vi "DiffOdometry_Update.vi"(6 "Reset Pose":T1={"TRANSLATION"={"X"=0.0, "Y"=0.0}, "ROTATION"={"VALUE"=0.0, "COS"=1.0, "SIN"=0.0}}, 8 "Reset":bool, 9 "Heading":T3={"VALUE"=0.0, "COS"=1.0, "SIN"=0.0}, 10 "RightDistance":dbl, 11 "LeftDistance":dbl) -> (3 "CurrentRelativePose":T1)   [LabVIEW 2019, in "Trajectory_Library.lvlib"]
doc: "SubVI for differential drive odometry. Odometry allows you to track the robot's position on the field over the course of a match using readings from 2 encoders and a gyroscope.\n\nTeams can use odometry during the autonomous period for complex tasks like path following. Furthermore, odometry can be used for latency compensation when using computer-vision systems.\n\nUpdates the robot position on the field using distance measurements from encoders. This method is more numerically accurate than using velocities to integrate the pose and is also advantageous for teams that are using lower CPR encoders.\n\nThis implementation slightly differs from the WPILIB C++/Java. The constructor, Update and Reset functions are incorporated into this single routine. There is no need to reset encoders or gyros. This routine compensates by remembering the values at reset. An optional \"Initial POSE\" can be specified to allow this routine to calculate absolute position. If not specified the position is relative to the position at reset. More than one instance of this can be used if needed. One instance could track absolute field position while another instance can track relative position for executing a trajectory.\n\nParameters:\n - Left distance -- Left wheel encoder distance (meters)\n - Right distance -- Right wheel encodeer distance (meters)\n - Heading - Robot gyroscope reading\n - Reset - When set, this resets the remembered left, right distance and gyroscope values, and sets the current pose to the initial pose. \n - Reset Pose - (Optional) When reset is TRUE this pose is used to set the current robot pose. (If the inital pose is zero or not present, the result will be a relative pose. If the reset pose is the absolute field pose, then the result current pose will be absolute.)\n\nResults:\n - currentRelativePose - The new pose of the robot. (If the initial pose is absolute, this will be an absolute pose.)"
uses:
  Trajectory_Library.lvlib
  POSE2D.ctl
  TRANSLATION2D.ctl
  ROTATION2D.ctl
  Rotation_UnaryMinus.vi
  Rotation_RotateBy.vi
  Rotation_CreateAngle.vi
  Rotation_CreateXY.vi
  Util_CalcDist.vi
  <vilib>/Rock Robotics/SystemInterfaces/NetworkCommunication/NetComm_UsageReport_ResourceType.ctl
  Util_LibraryGlobals.vi
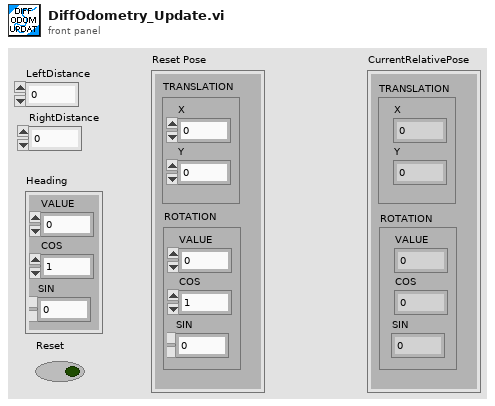
[diagram p1: front panel]
types:
  T1 = typedef "Trajectory_Library.lvlib/POSE2D.ctl" = cluster{"TRANSLATION":T2, "ROTATION":T3}
  T2 = typedef "Trajectory_Library.lvlib/TRANSLATION2D.ctl" = cluster{"X":dbl, "Y":dbl}
  T3 = typedef "Trajectory_Library.lvlib/ROTATION2D.ctl" = cluster{"VALUE":dbl, "COS":dbl, "SIN":dbl}
  T4 = typedef "NetComm_UsageReport_ResourceType.ctl" = enum8{"Controller", "Module", "Language", "CANPlugin", "Accelerometer", "ADXL345", "AnalogChannel", "AnalogTrigger", "AnalogTriggerOutput", "CANJaguar", "Compressor", "Counter", "Dashboard", "DigitalInput", "DigitalOutput", "DriverStationCIO", "DriverStationEIO", "DriverStationLCD", "Encoder", "GearTooth", "Gyro", "I2C", "Framework", "Jaguar", "Joystick", "Kinect", "KinectStick", "PIDController", "Preferences", "PWM", "Relay", "RobotDrive", "SerialPort", "Servo", "Solenoid", "SPI", "Task", "Ultrasonic", "Victor", "Button", "Command", "AxisCamera", "PCVideoServer", "SmartDashboard", "Talon", "HiTechnicColorSensor", "HiTechnicAccel", "HiTechnicCompass", "SRF08", "AnalogOutput", "Victor SP", "Talon SRX", "CAN Talon SRX", "ADXL362 Accel", "ADXRS450 Gyro", "Rev SPARK", "Mindsensors SD540", "Digital Filter", "ADIS16448", "PDP", "PCM", "PigeonIMU", "Nidec Brushless", "CTRE CANifier", "CTRE TalonFX", "CTRE Future 1", "CTRE Future 2", "CTRE Future 3", "CTRE Future 4", "CTRE Future 5", "CTRE Future 6", "Linear Filter", "Xbox Controller", "USB Camera", "NavX", "Pixy", "Pixy2", "ScanseSweep", "Shuffleboard", "CAN", "Digilent DMC60", "PWM Victor SPX", "Rev SPARK MAX PWM", "Rev SPARK MAX CAN", "ADIS16470", "PIDController2", "ProfiledPIDController", "Kinematics", "Odometry", "Units", "Trapezoid Profile", "DutyCycle", "Addressable LEDs", "Fusion Venom"}
  T5 = typedef "Trajectory_Library.lvlib/TWIST2D.ctl" = cluster{"dX":dbl, "dY":dbl, "dTHETA":dbl}
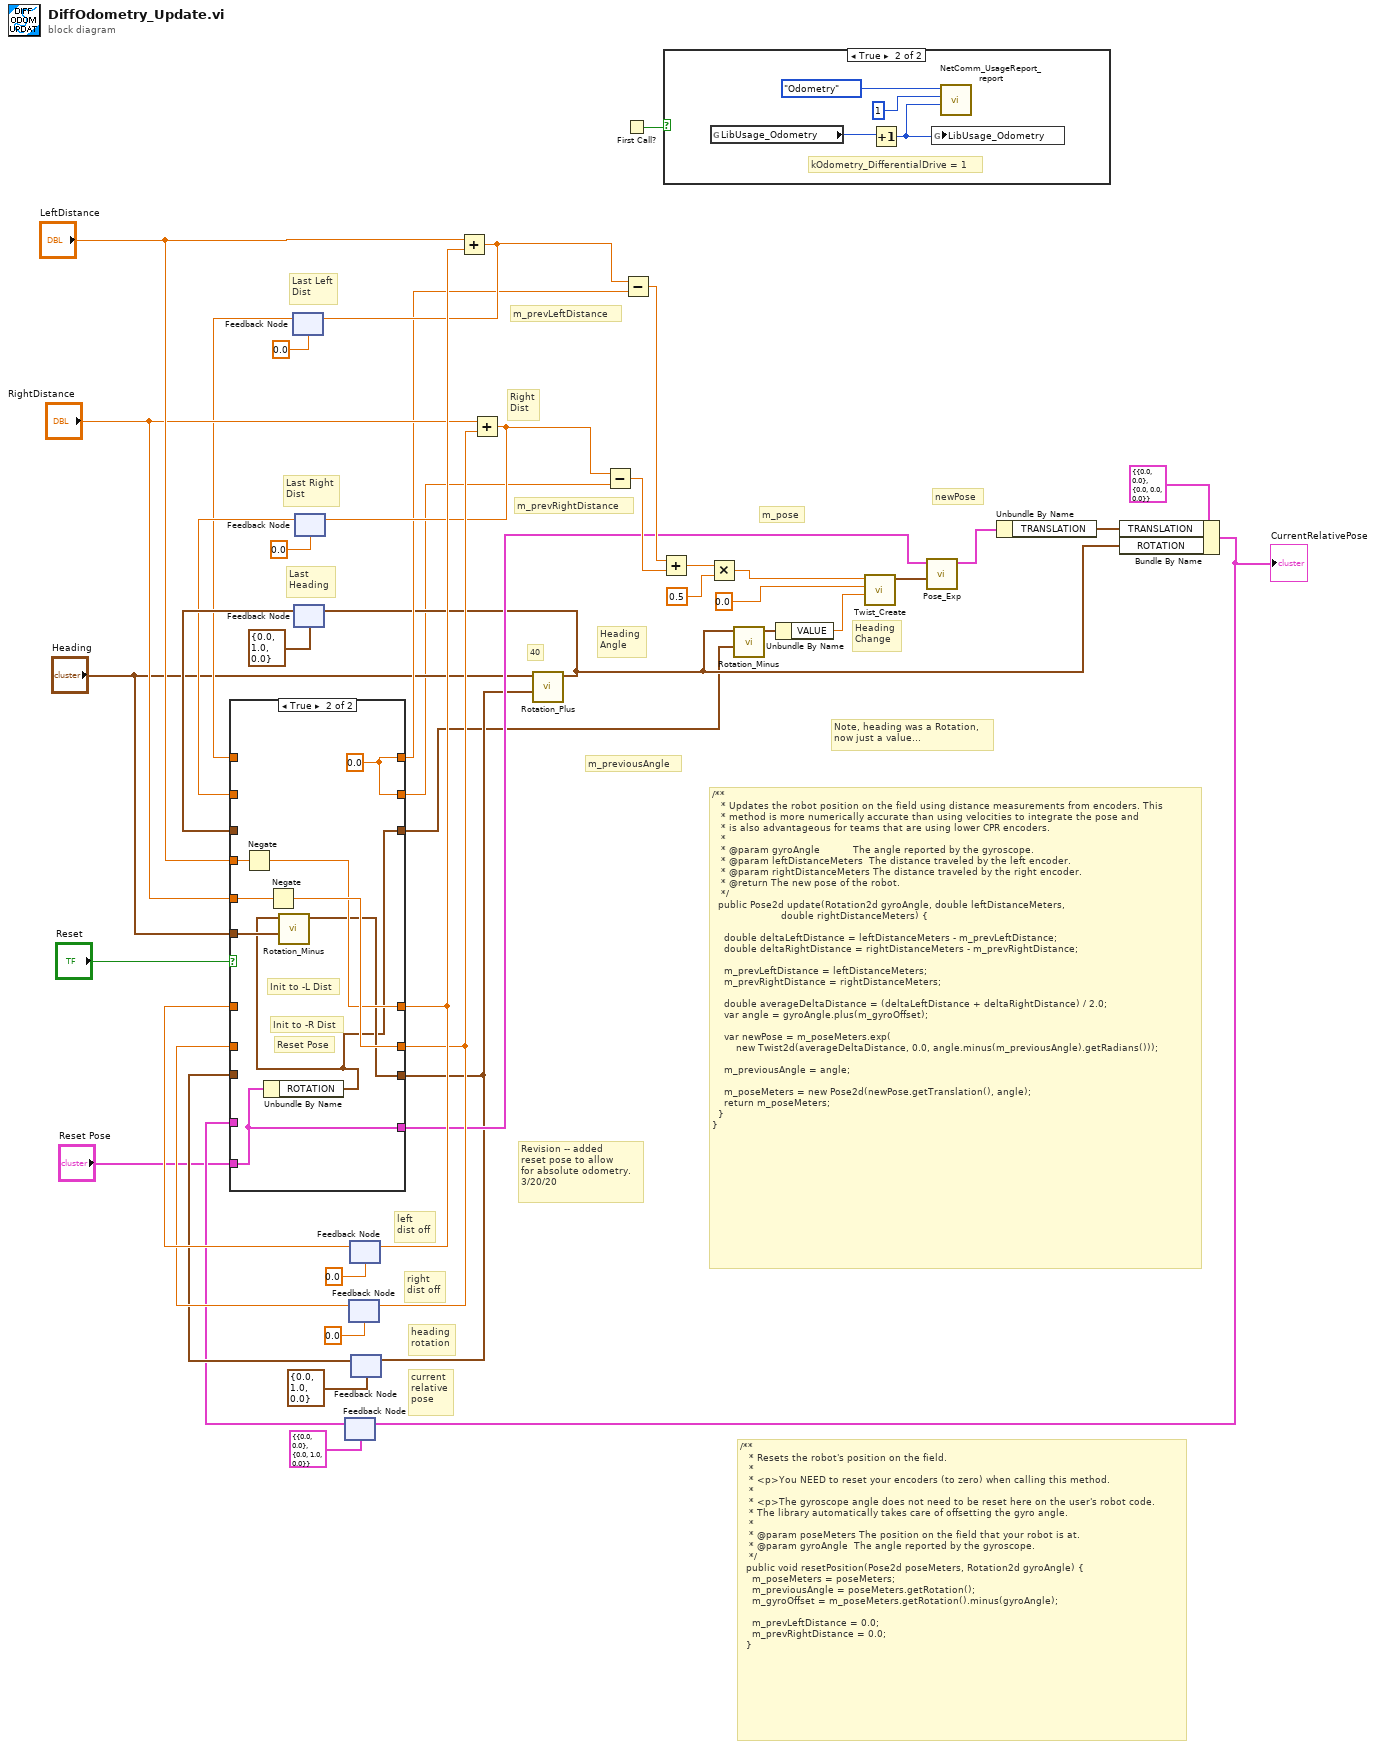
[diagram p0: block diagram]
diagram:
  # "Revision -- added\nreset pose to allow\nfor absolute odometry.\n3/20/20"
  # "40"
  # "left\ndist off"
  # "right\ndist off"
  # "heading\nrotation"
  # "current \nrelative\npose"
  # "/**\n   * Resets the robot's position on the field.\n   *\n   * <p>You NEED to reset your encoders (to zero) when calling this method.\n   *\n   * <p>The gyroscope angle does not need to be reset here on the user's robot code.\n   * The library automatically takes care of offsetting the gyro angle.\n   *\n   * @param poseMeters The position on the field that your robot is at.\n   * @param gyroAngle  The angle reported by the gyroscope.\n   */\n  public void resetPosition(Pose2d poseMeters, Rotation2d gyroAngle) {\n    m_poseMeters = poseMeters;\n    m_previousAngle = poseMeters.getRotation();\n    m_gyroOffset = m_poseMeters.getRotation().minus(gyroAngle);\n\n    m_prevLeftDistance = 0.0;\n    m_prevRightDistance = 0.0;\n  }"
  # "Heading\nChange"
  # "Note, heading was a Rotation,\nnow just a value..."
  # "Last\nHeading"
  # "Last Right\nDist"
  # "Last Left\nDist"
  # "Right\nDist"
  # "/**\n   * Updates the robot position on the field using distance measurements from encoders. This\n   * method is more numerically accurate than using velocities to integrate the pose and\n   * is also advantageous for teams that are using lower CPR encoders.\n   *\n   * @param gyroAngle           The angle reported by the gyroscope.\n   * @param leftDistanceMeters  The distance traveled by the left encoder.\n   * @param rightDistanceMeters The distance traveled by the right encoder.\n   * @return The new pose of the robot.\n   */\n  public Pose2d update(Rotation2d gyroAngle, double leftDistanceMeters,\n                       double rightDistanceMeters) {\n\n    double deltaLeftDistance = leftDistanceMeters - m_prevLeftDistance;\n    double deltaRightDistance = rightDistanceMeters - m_prevRightDistance;\n\n    m_prevLeftDistance = leftDistanceMeters;\n    m_prevRightDistance = rightDistanceMeters;\n\n    double averageDeltaDistance = (deltaLeftDistance + deltaRightDistance) / 2.0;\n    var angle = gyroAngle.plus(m_gyroOffset);\n\n    var newPose = m_poseMeters.exp(\n        new Twist2d(averageDeltaDistance, 0.0, angle.minus(m_previousAngle).getRadians()));\n\n    m_previousAngle = angle;\n\n    m_poseMeters = new Pose2d(newPose.getTranslation(), angle);\n    return m_poseMeters;\n  }\n}"
  # "newPose"
  # "Heading\nAngle"
  # "m_prevRightDistance"
  # "m_prevLeftDistance"
  # "m_previousAngle"
  # "m_pose"
  n1 = feedback #1(0.0 ("LeftDistance")) -> (w16:dbl)
  n2 = feedback #2(T3 {"VALUE"=0.0, "COS"=1.0, "SIN"=0.0} ("ROTATION")) -> (w19:T3)
  n3 = feedback #3(0.0 ("RightDistance")) -> (w18:dbl)
  n4 = feedback #4(T1 {"TRANSLATION"={"X"=0.0, "Y"=0.0}, "ROTATION"={"VALUE"=0.0, "COS"=1.0, "SIN"=0.0}} ("POSE")) -> (w21:T1)
  n5 = feedback #5(0.0 ("LeftDistance")) -> (w35:dbl)
  n6 = feedback #6(0.0 ("LeftDistance")) -> (w36:dbl)
  n7 = feedback #7(T3 {"VALUE"=0.0, "COS"=1.0, "SIN"=0.0} ("ROTATION")) -> (w34:T3)
  n8 = case shown="True" "Reset" {
    tunnel: "Heading" -> [_ w54]
    tunnel: "RightDistance" -> [_ w58]
    tunnel: "LeftDistance" -> [_ w59]
    tunnel: [w50 w56] -> w30
    tunnel: [w49 w57] -> w26
    tunnel: [w48 w55] -> w6
    tunnel: w36 -> [w50 _]
    tunnel: w35 -> [w49 _]
    tunnel: w34 -> [w48 _]
    tunnel: [w47 w51] -> w20
    tunnel: w21 -> [w47 _]
    tunnel: w19 -> [w46 _]
    tunnel: [w46 w53] -> w4
    tunnel: w18 -> [w45 _]
    tunnel: [w45 w52] -> w3
    tunnel: [w44 w52] -> w17
    tunnel: w16 -> [w44 _]
    tunnel: "Reset Pose" -> [_ w51]
    frame False {
      # "Last Left Dist"
      # "Last Right Dist"
      # "Last Heading"
      # "(-) Left Dist at Reset"
      # "(-) Right Dist at Reset"
      # "Heading at Reset"
      # "Saved Relative POSE"
    }
    frame True {
      w52 = 0.0 ("LeftDistance")
      # "Init to -L Dist"
      # "Init to -R Dist"
      # "Reset Pose"
      n9 = Negate(x=w59) -> (-x=w56:dbl)
      n10 = Unbundle By Name(w51) -> ("ROTATION"=w53:T3)
      n11 = Negate(x=w58) -> (-x=w57:dbl)
      n12 = call "Rotation_Minus.vi"("other ROTATION"=w54, "in ROTATION"=w53) -> ("out ROTATION"=w55:T3)  [unwired: 9 in]
    }
  }
  n13 = feedback-in #5(w26) -> ()
  n14 = feedback-in #6(w30) -> ()
  n15 = feedback-in #7(w6) -> ()
  n16 = Add(x="LeftDistance", y=w30) -> (x+y=w28:dbl)
  n17 = feedback-in #1(w28) -> ()
  n18 = Add(x="RightDistance", y=w26) -> (x+y=w25:dbl)
  n19 = feedback-in #3(w25) -> ()
  n20 = call "Rotation_Plus.vi"("other ROTATION"=w6, "in ROTATION"="Heading") -> ("out ROTATION"=w5:T3)  [unwired: 9 in]
  n21 = feedback-in #2(w5) -> ()
  n22 = Subtract(x=w25, y=w3) -> (x-y=w42:dbl)
  n23 = First Call?() -> (First Call?: T/F=w1:bool)
  n24 = Subtract(x=w28, y=w17) -> (x-y=w43:dbl)
  n25 = Add(x=w43, y=w42) -> (x+y=w41:dbl)
  n26 = case shown="True" w1 {
    frame False {
    }
    frame True {
      # "kOdometry_DifferentialDrive = 1"
      n27 = global read "Util_LibraryGlobals.vi" "LibUsage_Odometry"() -> (w62:i32)
      n28 = Increment(x=w62) -> (x+1=w61:i32)
      n29 = global write "Util_LibraryGlobals.vi" "LibUsage_Odometry"(w61) -> ()
      n30 = call <vilib>:"NetComm_UsageReport_report.vi"("Context"=w61, "Instance Number"=u8 1, "Resource Type"=NetComm_UsageReport_ResourceType."Odometry") -> ()  [unwired: 9 in]
    }
  }
  n31 = Multiply(x=w41, y=0.5) -> (x*y=w24:dbl)
  n32 = call "Rotation_Minus.vi"("other ROTATION"=w4, "in ROTATION"=w5) -> ("out ROTATION"=w11:T3)  [unwired: 9 in]
  n33 = Unbundle By Name(w11) -> ("VALUE"=w10:dbl)
  n34 = call "Twist_Create.vi"("dTHETA"=w10, "dY"=0.0 ("DeltaY"), "dX"=w24) -> ("TWIST"=w22:T5)  [unwired: 8 in]
  n35 = call "Pose_Exp.vi"("TWIST"=w22, "POSE"=w20) -> ("UpdatedPose"=w15:T1)  [unwired: 9 in]
  n36 = Unbundle By Name(w15) -> ("TRANSLATION"=w13:T2)
  n37 = Bundle By Name(cluster=T1 {"TRANSLATION"={"X"=0.0, "Y"=0.0}, "ROTATION"={"VALUE"=0.0, "COS"=0.0, "SIN"=0.0}} ("POSE"), "TRANSLATION"=w13, "ROTATION"=w5) -> (w12:T1)
  "CurrentRelativePose" <- w12
  n38 = feedback-in #4(w12) -> ()
